vi "SLSC Create Properties Section.vi"(0 "Parent Ref in":T2 format="%.0x", 1 "GUID Properties Root Page":string, 2 "GUID Get Properties Page":string, 3 "GUID Set Properties Page":string, 5 "Properties":string, 7 "Physical Channel":string, 9 "properties":T3[](array[typedef]), 11 "error in (no error)":errorcluster, 12 "enums":T1[](array[typedef]), 13 "SLSCChannelPath":string, 14 "Documentation":string) -> (4 "Parent Ref out":T2 format="%.0x", 15 "error out":errorcluster)   [LabVIEW 2017, in "SLSC CD System Explorer.lvlib"]
uses:
  SLSC CD System Explorer.lvlib
  SLSC EDS API/JSON parsing/property.ctl
  <vilib>/NI Veristand/Custom Device API/Custom Device Item Ref.ctl
  SLSC EDS API/JSON parsing/enum.ctl
  <vilib>/NI VeriStand/Custom Device API/Custom Device API.lvlib
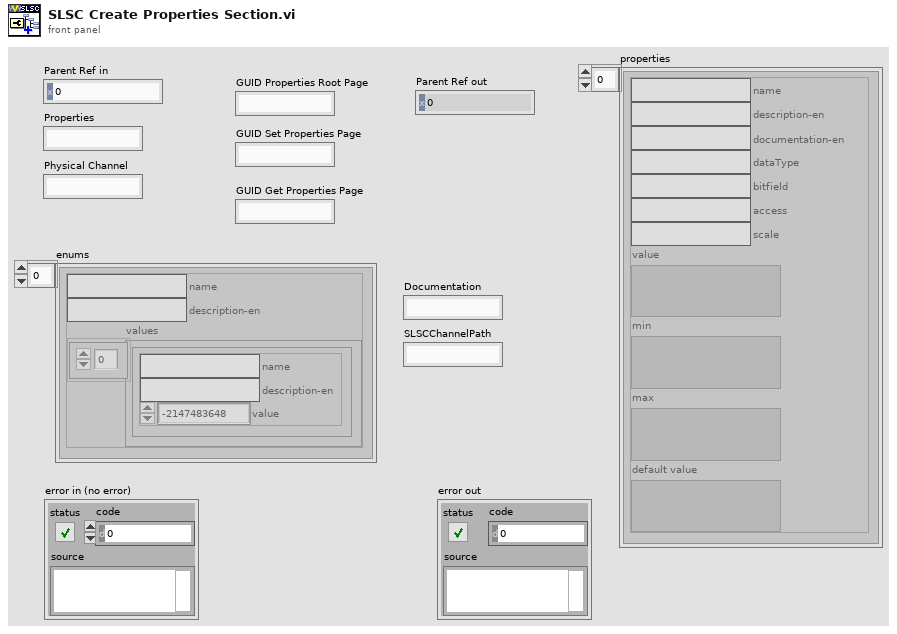
[diagram p1: front panel]
types:
  T1 = typedef "enum.ctl" = cluster{"name":string, "description-en":string, "values":cluster{"name":string, "description-en":string, "value":i32}[]}
  T2 = typedef "Custom Device API.lvlib/Custom Device Item Ref.ctl" = u64
  T3 = typedef "property.ctl" = cluster{"name":string, "description-en":string, "documentation-en":string, "dataType":string, "bitfield":string, "access":string, "scale":string, "value":variant, "min":variant, "max":variant, "default value":variant}
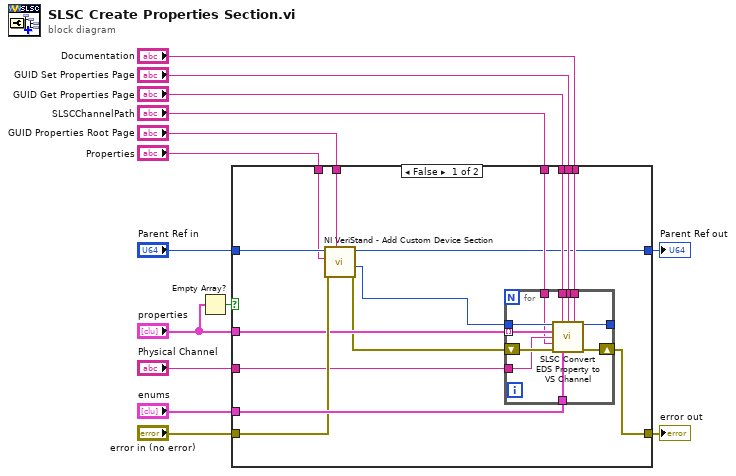
[diagram p0: block diagram]
diagram:
  n1 = Empty Array?(array="properties") -> (empty?=w14:bool)
  n2 = case shown="False" w14 {
    tunnel: [w29 w41] -> w1
    tunnel: "GUID Get Properties Page" -> [w28 _]
    tunnel: "Documentation" -> [w27 _]
    tunnel: "SLSCChannelPath" -> [w26 _]
    tunnel: "enums" -> [w25 _]
    tunnel: "GUID Set Properties Page" -> [w24 _]
    tunnel: [w23 w42] -> w7
    tunnel: "Parent Ref in" -> [w22 w42]
    tunnel: "error in (no error)" -> [w21 w41]
    tunnel: "Properties" -> [w20 _]
    tunnel: "GUID Properties Root Page" -> [w19 _]
    tunnel: "Physical Channel" -> [w18 _]
    tunnel: "properties" -> [w17 _]
    frame False {
      n3 = call <vilib>:"NI VeriStand - Add Custom Device Section.vi"("GUID (Default Section)"=w19, "error in (no error)"=w21, "Section Name"=w20, "Parent Ref in"=w22) -> ("error out"=w16:errorcluster, "Section Ptr"=w15:T2, "Parent Ref out"=w23:T2)  [unwired: 4 in, 1 out]
      n4 = for {
        shift-right: [w38] -> w29
        shift-left: w16 -> [w40]
        tunnel: w17 -> [w36] mode=indexing
        tunnel: w24 -> [w31]
        tunnel: w26 -> [w32]
        tunnel: w27 -> [w35]
        tunnel: w18 -> [w33]
        tunnel: w25 -> [w34]
        tunnel: w28 -> [w30]
        tunnel: w15 -> [w37]
        tunnel: [w39] -> _
        n5 = call "SLSC Convert EDS Property to VS Channel.vi"("Section Ptr"=w37, "GUID Get Properties Page"=w30, "GUID Set Properties Page"=w31, "Documentation"=w35, "property"=w36, "Physical Channel"=w33, "SLSCChannelPath"=w32, "error in (no error)"=w40, "enums"=w34) -> ("Parent Ref out"=w39:T2, "error out"=w38:errorcluster)  [unwired: 5 in]
      }
    }
    frame True {
    }
  }
  "Parent Ref out" <- w7
  "error out" <- w1
